vi "ProdaNG.Languages.Get.vi"(8 "error in (no error)":errorcluster, 11 "dbHandleIn":i32) -> (0 "error out":errorcluster, 2 "Languages":T1[](array[typedef]), 3 "dbHandle":i32)   [LabVIEW 2016]
doc: "This function returns a product structure for a product, which is identified by a part and a serial number.\nImportant information: The field 'individual' was taken over from the field 'allgemein' of the legacy data directly. Because of this most products have the value 0 further on and only a few the value 1. \nParameter:\nhandle is an Integer, which is returned by the function Login() at the creation of a new connection.\nwabcoPartId is the Id of the part.\nserialNumber is the serial number of the product for the part above.\nproduct is a pointer on a product structure, which is filled if the returncode is 0. The structure must be defined in the calling program.\n\nReturncodes:\n0 No error\n< 0 ORACLE Error code\n6 (ERROR_INVALID_HANDLE) in case of an invalid handle\n1403 Record does not exist"
uses:
  Controls/ProdaNG.Language.ctl
  Controls/ProdaNG.LanguageSize.ctl
  <vilib>/Utility/importsl/GetValueByPointer/datatype.ctl
  <vilib>/Utility/importsl/GetValueByPointer/GetValueByPointer.xnode
  prodllNG.dll
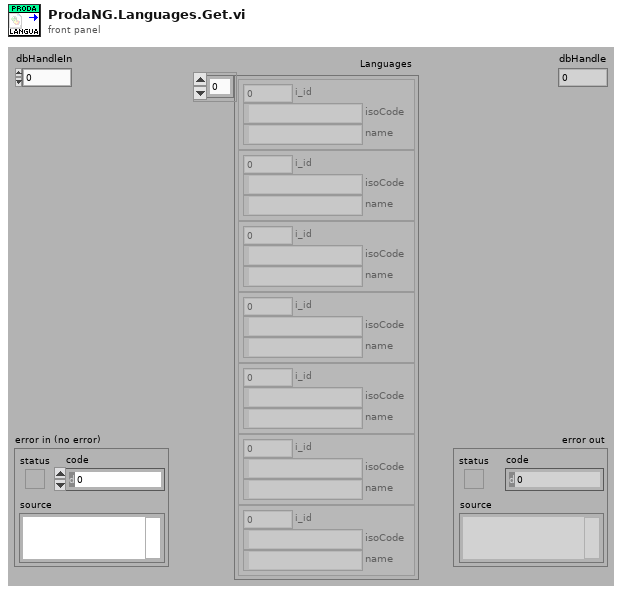
[diagram p1: front panel]
types:
  T1 = typedef "ProdaNG.Language.ctl" = cluster{"i_id":i32, "isoCode":string, "name":string}
  T2 = typedef "ProdaNG.LanguageSize.ctl" = cluster{"i_id":i32, "isoCode":i32, "name":i32}
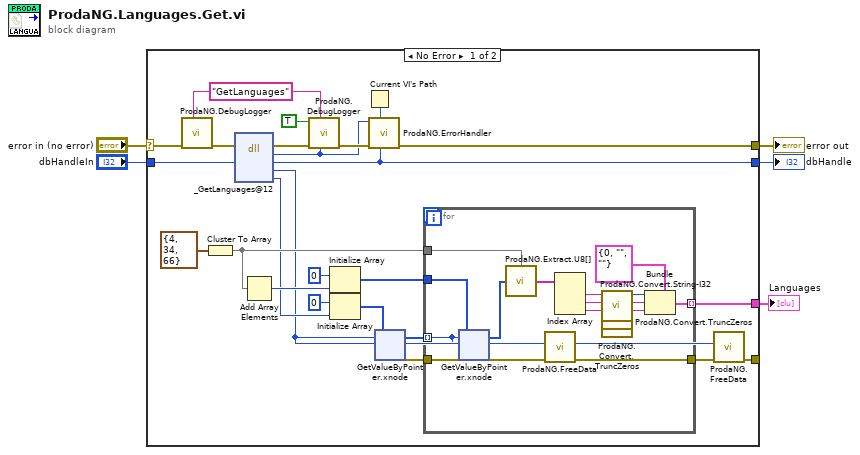
[diagram p0: block diagram]
diagram:
  n1 = case shown="No Error" "error in (no error)" {
    selector: "error in (no error)" -> [w26 w78]
    tunnel: "dbHandleIn" -> [w28 w77]
    tunnel: [w29 w77] -> w3
    tunnel: [w10 _] -> w2
    tunnel: [w9 w78] -> w1
    tunnel: [w6 _] -> _
    frame No Error {
      w22 = "GetLanguages" ("cmd")
      n2 = call "ProdaNG.DebugLogger.vi"("cmd"=w22, "error in (no error)"=w26) -> ("error out"=w25:errorcluster)  [unwired: 9 in]
      n3 = Cluster To Array(cluster=T2 {"i_id"=4, "isoCode"=34, "name"=66} ("LanguageSize")) -> (array=w14:i32[])
      n4 = dll-call lib="D:/Maszup/WABCO/SVN/LineTraceSystem/SOFTWARE/sources/Database/ProdaNG/prodllNG.dll" fn="_GetLanguages@12" ("ProDLL wrapper.dll:ProDLL_wrapper_GetWabcoParts_GetData")(error in=w25, "dbHandle"=w28) -> (error out=w24:errorcluster, "return type"=w21:i32, "dbHandle"=w29:i32, "languages"=w7:u32, "countPtr"=w11:i32)  [unwired: 4 in, 1 out]
      n5 = Add Array Elements(numeric array=w14) -> (sum=w15:i32)
      n6 = call "ProdaNG.DebugLogger.vi"("return type"=w21, "cmd"=w22, "error in (no error)"=w24, "done? (F)"=TRUE) -> ("error out"=w23:errorcluster)  [unwired: 7 in]
      n7 = Initialize Array(u8 0 ("element"), w15) -> (w16:u8[])
      n8 = Initialize Array(u32 0 ("element"), w11) -> (w20:u32[])
      n9 = Current VI's Path() -> (path=w30:path)
      n10 = call "ProdaNG.ErrorHandler.vi"("dbHandleIn"=w29, "Path"=w30, "error in"=w23, "output_parameter"=w21) -> ("error out"=w9:errorcluster)  [unwired: 7 in]
      n11 = xnode "GetValueByPointer.xnode"("Pointer"=w7, "InputType"=w20) -> ("Output"=w12:u32[], "ErrorOut"=w18:errorcluster)  [unwired: 2 in]
      n12 = for {
        tunnel: w18 -> [w46]
        tunnel: w12 -> [w33] mode=indexing
        tunnel: w16 -> [w45]
        tunnel: w14 -> [w39]
        tunnel: [w38] -> w10 mode=indexing
        tunnel: [w32] -> w8
        n13 = xnode "GetValueByPointer.xnode"("Pointer"=w33, "InputType"=w45, "ErrorIn"=w46) -> ("Output"=w41:u8[], "ErrorOut"=w31:errorcluster)  [unwired: 1 in]
        n14 = call "ProdaNG.Extract.U8[].vi"("unsigned byte array"=w41, "Sizes"=w39) -> ("Elements"=w40:string[])
        n15 = call "ProdaNG.FreeData.vi"("error in (no error)"=w31, "Pointers"=w33) -> ("error out"=w32:errorcluster)  [unwired: 9 in]
        n16 = Index Array(array=w40) -> (element #1=w42:string, element #2=w36:string, element #3=w35:string)  [unwired: 3 in]
        n17 = call "ProdaNG.Convert.String-I32.vi"("unsigned byte string"=w42) -> ("32bit integer"=w43:i32)  [unwired: 10 in]
        n18 = call "ProdaNG.Convert.TruncZeros.vi"("string with \\0s"=w36) -> ("LV string"=w37:string)  [unwired: 10 in]
        n19 = call "ProdaNG.Convert.TruncZeros.vi"("string with \\0s"=w35) -> ("LV string"=w34:string)  [unwired: 10 in]
        n20 = Bundle(cluster=T1 {"i_id"=0, "isoCode"="", "name"=""} ("Language"), "i_id"=w43, "isoCode"=w37, "name"=w34) -> (w38:T1)
      }
      n21 = call "ProdaNG.FreeData.vi"("error in (no error)"=w8, "Pointers"=w7) -> ("error out"=w6:errorcluster)  [unwired: 9 in]
    }
    frame Error {
    }
  }
  "error out" <- w1
  "dbHandle" <- w3
  "Languages" <- w2
